vi "temp chart with power BAE7.vi"(1 "exit T control":bool, 7 "Control Parameters":T4={"Setpoint"=50.0, "Control bandwidth"=4.0, "Settle bandwidth"=1.0} {"Settle bandwidth" format="%.2f"; "Control bandwidth" format="%.2f"; "Setpoint" format="%.2f"}, 11 "error in":errorcluster) -> (8 "Temp":dbl format="%.2f", 15 "error out":errorcluster)   [LabVIEW 2014]
doc: "temp chart with power BAE7\n\nIn run time records, plots, and displays how the temperature of a \"bug,\" an assortment of a capacitor, thermistor, and resistor is affected by normalized power. This uses ELVIS II multimeter as the measuring device. \n\nBeverly Abadines\nPHY 350\nE7"
panel:
  in  "Scale Control":T1
  in  "Power Control":dbl(slide) scale=0.0..1.0
  out "range indicators":T2={"In control band"=FALSE, "In settle band"=FALSE, "under range"=TRUE, "over range"=FALSE}
  out "Power":dbl=0.754407202908737 format="%.2f"
  out "Setpoint":dbl=50.0 format="%.2f"
  out "Temperature History":T3(graph)={"temp out"=29.702811899974034, 50.0, 50.5, 49.5, 50.1, 49.9, 50.508814405817475}
  # "Manual Temperature Controller"
  # "1.0"
  # "Norm\nPower\nscale"
  # "0.5"
  # "0.0"
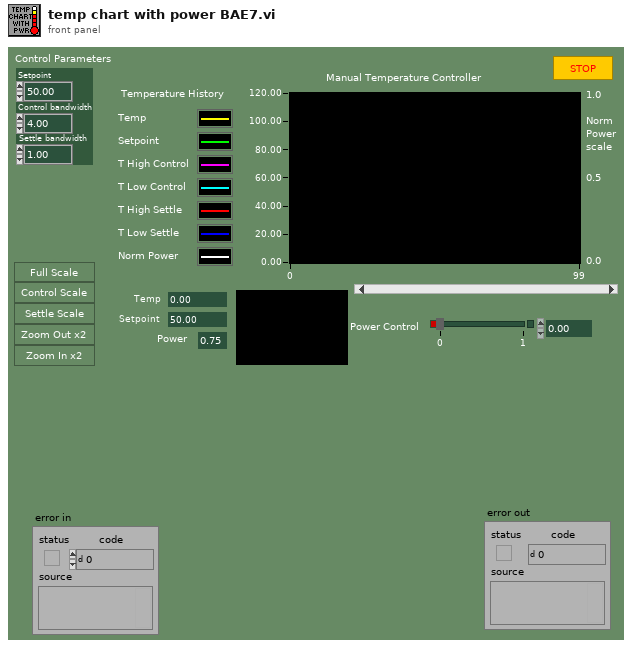
[diagram p1: front panel]
types:
  T1 = cluster{"Full Scale":bool, "Control Scale":bool, "Settle Scale":bool, "Zoom Out":bool, "Zoom In":bool}
  T2 = cluster{"In control band":bool, "In settle band":bool, "under range":bool, "over range":bool}
  T3 = cluster{"temp out":dbl, dbl, dbl, dbl, dbl, dbl, dbl}
  T4 = cluster{"Setpoint":dbl, "Control bandwidth":dbl, "Settle bandwidth":dbl}
  T5 = cluster{"[0]":refnum<vi>, "[1]":refnum<vi>, "[2]":refnum<vi>, "[3]":refnum<vi>}
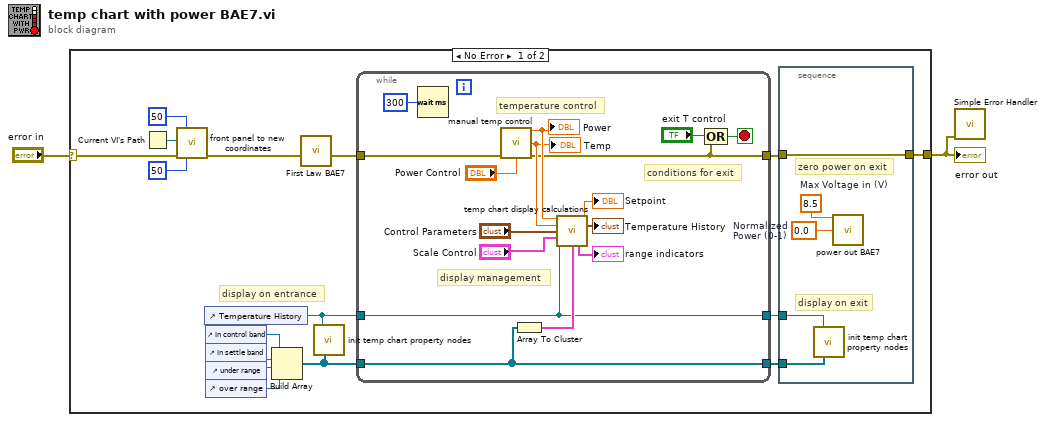
[diagram p0: block diagram]
diagram:
  n1 = case shown="No Error" "error in" {
    selector: "error in" -> [w9 w40]
    tunnel: [w5 w40] -> w1
    frame No Error {
      # "display on entrance"
      n2 = Current VI's Path() -> (path=w6:path)
      n3 = call "front panel to new coordinates.vi"("new top"=i16 50, "path"=w6, "error in (no error)"=w9, "new left"=i16 50) -> ("error out"=w4:errorcluster)  [unwired: 11 in]
      n4 = control-ref of="Temperature History"() -> (w16:refnum<vi>)
      n5 = control-ref of="In control band"() -> (w10:refnum<vi>)
      n6 = control-ref of="In settle band"() -> (w11:refnum<vi>)
      n7 = control-ref of="under range"() -> (w12:refnum<vi>)
      n8 = control-ref of="over range"() -> (w13:refnum<vi>)
      n9 = Build Array(w10, w11, w12, w13) -> (w17:refnum<vi>[])
      n10 = call "First Law BAE7.vi"("error in"=w4) -> ("error out"=w3:errorcluster)  [unwired: 8 in]
      n11 = call "init temp chart property nodes.vi"("Temperature History"=w16, "range indicators"=w17) -> ()  [unwired: 3 in, 11 out]
      n12 = while {
        tunnel: [w25] -> w14
        tunnel: [w26] -> w15
        tunnel: w16 -> [w25]
        tunnel: w17 -> [w26]
        tunnel: w3 -> [w19]
        tunnel: [w20] -> w18
        stop <- w28 stop-if-true
        # "display management"
        # "conditions for exit"
        # "temperature control"
        n13 = Wait (ms)(milliseconds to wait=u32 300) -> ()  [unwired: 1 out]
        n14 = call "manual temp control.vi"("error in"=w19, "Normalized Power In (0-1)"="Power Control") -> ("power meas (0-1)"=w24:dbl, "temp meas"=w23:dbl, "error out"=w20:errorcluster)  [unwired: 4 in, 7 out]
        "Temp" <- w23
        "Power" <- w24
        n15 = Array To Cluster(array=w26) -> (cluster=w27:T5)
        n16 = call "temp chart display calculations.vi"("power in (0-1)"=w24, "temp in"=w23, "Control Parameters"="Control Parameters", "Scale Control In"="Scale Control", "Temp History in"=w25, "range indicators"=w27) -> ("Setpoint out"=→"Setpoint":dbl, "Temperature History out"=→"Temperature History":T3, "range indicators out"=→"range indicators":T2)  [unwired: 3 in, 4 out]
        n17 = Compound Arithmetic op=OR("exit T control", w20) -> (w28:bool)
      }
      n18 = stacked-sequence {
        tunnel: [w35] -> w5
        tunnel: w18 -> [w35]
        tunnel: w15 -> [w39]
        tunnel: w14 -> [w38]
        frame #0 {
          w37 = 8.5  # Max Voltage in (V)
          w36 = 0.0  # Normalized Power (0-1)
          # "display on exit"
          # "zero power on exit"
          n19 = call "init temp chart property nodes.vi"("Temperature History"=w38, "range indicators"=w39) -> ()  [unwired: 4 in, 10 out]
          n20 = call "power out BAE7.vi"("Max Voltage in (V)"=w37, "Normalized Power (0-1)"=w36) -> ()  [unwired: 12 in, 2 out]
        }
      }
    }
    frame Error {
    }
  }
  "error out" <- w1
  n21 = call <vilib>:"Simple Error Handler.vi"("error in (no error)"=w1) -> ()  [unwired: 4 in, 5 out]
